vi "Set PC Settings (Keith Koch's conflicted copy 2013-05-10).vi"   [LabVIEW 2011]
uses:
  _GlobalVariables&Libraries/ATV Program Global Variables.vi
types:
  T1 = cluster{"End ATV Program":bool, "E-Stop":bool, "Save Logfile":bool, "Logfile Iteration Delay (ms)":u32, "Loop iteration time (ms)":u32, "Logfile Location":path, "Default GPS Navigation Path":path, "Computer":string, "Default GPS Boundary Path":path}
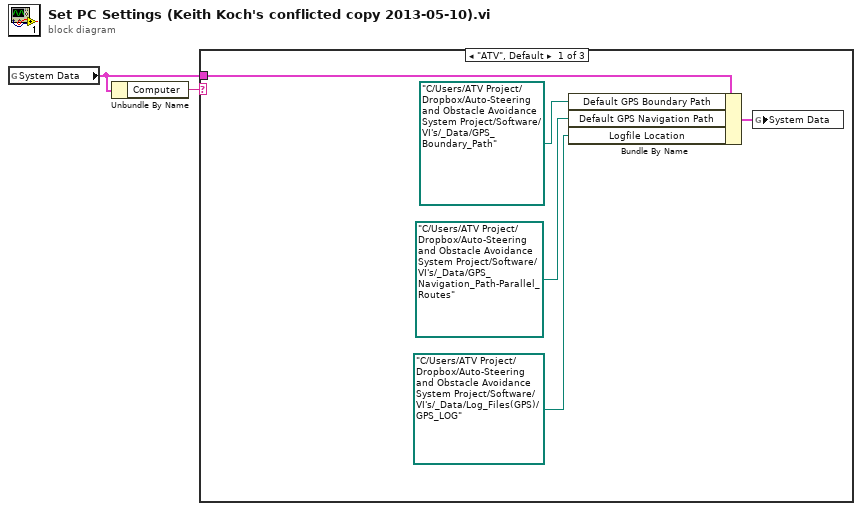
[diagram p0: block diagram]
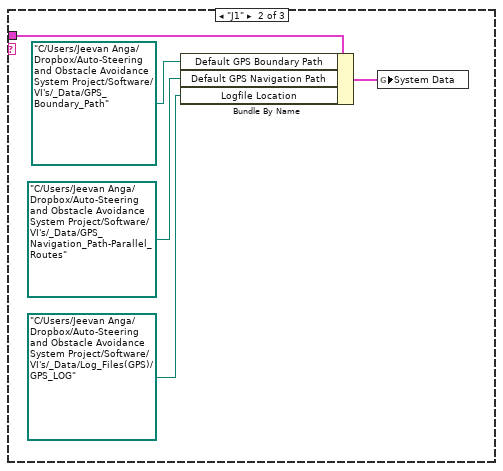
[diagram p2: hidden frame]
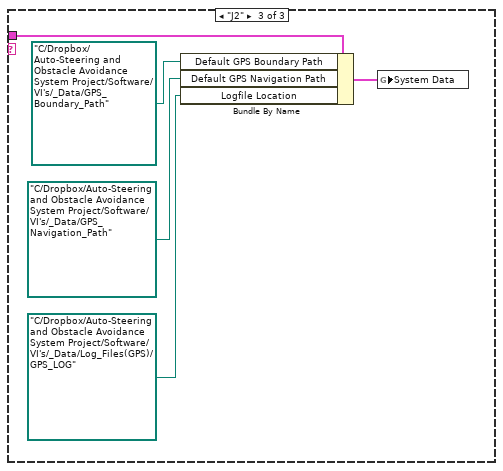
[diagram p3: hidden frame]
diagram:
  n1 = global read "ATV Program Global Variables.vi" "System Data"() -> (w1:T1)
  n2 = Unbundle By Name(w1) -> ("Computer"=w2:string)
  n3 = case shown="\"ATV\", Default" w2 {
    tunnel: w1 -> [w7 w10 w14]
    frame "ATV", Default {
      n4 = Bundle By Name(cluster=w7, "Default GPS Boundary Path"=path "C:/Users/ATV Project/Dropbox/Auto-Steering and Obstacle Avoidance System Project/Software/VI's/_Data/GPS_Boundary_Path", "Default GPS Navigation Path"=path "C:/Users/ATV Project/Dropbox/Auto-Steering and Obstacle Avoidance System Project/Software/VI's/_Data/GPS_Navigation_Path-Parallel_Routes", "Logfile Location"=path "C:/Users/ATV Project/Dropbox/Auto-Steering and Obstacle Avoidance System Project/Software/VI's/_Data/Log_Files(GPS)/GPS_LOG" ("Default GPS Navigation Path")) -> (w5:T1)
      n5 = global write "ATV Program Global Variables.vi" "System Data"(w5) -> ()
    }
    frame "J1" {
      n6 = Bundle By Name(cluster=w10, "Default GPS Boundary Path"=path "C:/Users/Jeevan Anga/Dropbox/Auto-Steering and Obstacle Avoidance System Project/Software/VI's/_Data/GPS_Boundary_Path", "Default GPS Navigation Path"=path "C:/Users/Jeevan Anga/Dropbox/Auto-Steering and Obstacle Avoidance System Project/Software/VI's/_Data/GPS_Navigation_Path-Parallel_Routes", "Logfile Location"=path "C:/Users/Jeevan Anga/Dropbox/Auto-Steering and Obstacle Avoidance System Project/Software/VI's/_Data/Log_Files(GPS)/GPS_LOG" ("Default GPS Navigation Path")) -> (w11:T1)
      n7 = global write "ATV Program Global Variables.vi" "System Data"(w11) -> ()
    }
    frame "J2" {
      n8 = Bundle By Name(cluster=w14, "Default GPS Boundary Path"=path "C:/Dropbox/Auto-Steering and Obstacle Avoidance System Project/Software/VI's/_Data/GPS_Boundary_Path", "Default GPS Navigation Path"=path "C:/Dropbox/Auto-Steering and Obstacle Avoidance System Project/Software/VI's/_Data/GPS_Navigation_Path", "Logfile Location"=path "C:/Dropbox/Auto-Steering and Obstacle Avoidance System Project/Software/VI's/_Data/Log_Files(GPS)/GPS_LOG" ("Default GPS Navigation Path")) -> (w16:T1)
      n9 = global write "ATV Program Global Variables.vi" "System Data"(w16) -> ()
    }
  }
